vi "Add Item to Tree.vi"(6 "Display Text Override":string, 7 "Child only? (F)":bool, 8 "error in (no error)":errorcluster, 9 "Parent Tag":string, 10 "Data Item":refnum<class "Data Item.lvclass">, 11 "Tree Manager in":refnum<class "Tree Manager.lvclass">) -> (0 "error out":errorcluster, 2 "New Tag":string, 3 "Tree Manager out":refnum<class "Tree Manager.lvclass">)   [LabVIEW 2023, in "VILab.lvlib" / "Tree Manager.lvclass"]
uses:
  Tree Manager.lvclass
  Data Item.lvclass
  Tree Manager.lvclass/Tree Manager.ctl
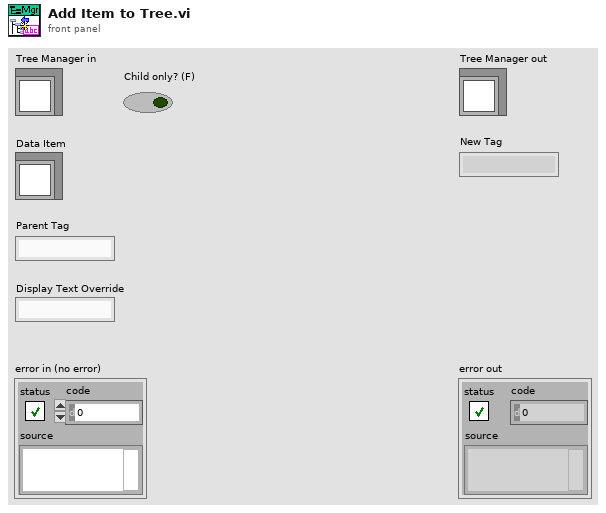
[diagram p1: front panel]
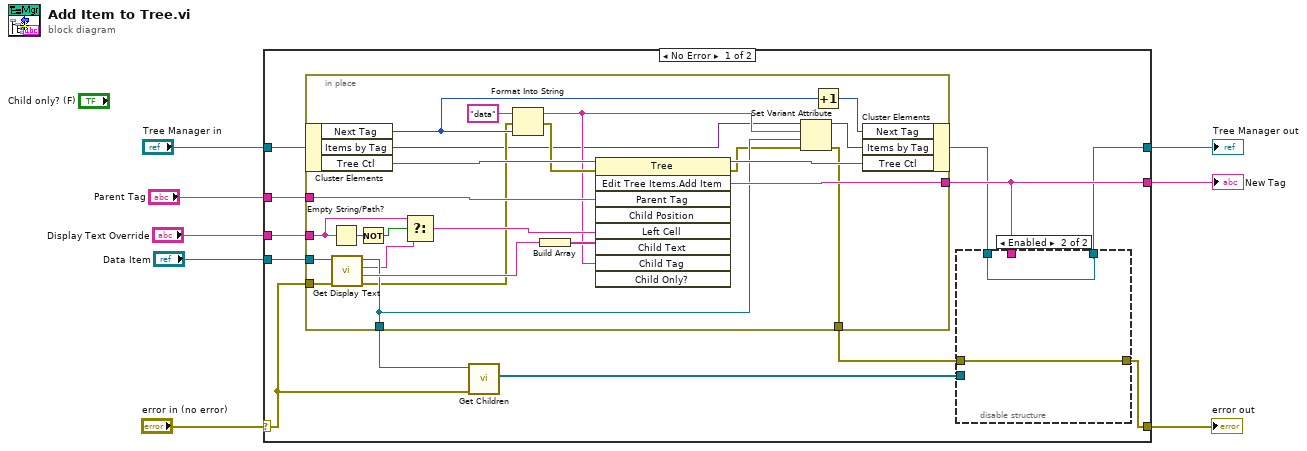
[diagram p0: block diagram]
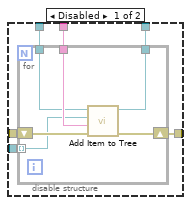
[diagram p2: hidden frame]
diagram:
  n1 = case shown="No Error" "error in (no error)" {
    selector: "error in (no error)" -> [w16 w60]
    tunnel: [w10 w60] -> w7
    tunnel: [w12 w59] -> w5
    tunnel: "Tree Manager in" -> [w19 w59]
    tunnel: "Data Item" -> [w20 _]
    tunnel: "Parent Tag" -> [w18 _]
    tunnel: [w15 _] -> w2
    tunnel: "Display Text Override" -> [w9 _]
    frame No Error {
      n2 = in-place {
        in-place-border: w20 -> [w58]
        in-place-border: w16 -> [w57]
        in-place-border: w18 -> [w55]
        in-place-border: [w47] -> w15
        in-place-border: [w46] -> w14
        in-place-border: [w45] -> w17
        in-place-border: w9 -> [w42]
        n3 = in-place-cluster #1(w19) -> ("Next Tag"=w49:u64, "Items by Tag"=w35:variant, "Tree Ctl"=w56:refnum<vi>)
        n4 = Empty String/Path?(string/path=w42) -> (empty?=w44:bool)
        n5 = call-dynamic "Get Display Text.vi"("error in (no error)"=w57, "Data Item in"=w58) -> ("error out"=w39:errorcluster, "Detail Text"=w54:string, "Display Name"=w41:string, "Data Item out"=w45:refnum<class "Data Item.lvclass">)  [unwired: 6 in]
        n6 = Not(x=w44) -> (.not. x?=w43:bool)
        n7 = Select(t=w42, s=w43, f=w41) -> (s? t:f=w40:string)
        n8 = Format Into String(initial string="data", error in=w39, w49) -> (resulting string=w36:string, error out=w38:errorcluster)  [unwired: 1 in]
        n9 = Build Array(w54) -> (w53:string[])
        n10 = invoke class="Tree" method="Edit Tree Items.Add Item"(reference=w56, error in=w38, "Parent Tag"=w55, "Left Cell"=w40, "Child Text"=w53, "Child Tag"=w36) -> (reference out=w52:refnum<vi>, error out=w37:errorcluster, "Edit Tree Items:Add Item"=w47:string)  [unwired: 3 in, 6 out]
        n11 = Set Variant Attribute(Variant=w35, name=w36, value=w45, error in=w37) -> (Variant out=w51:variant, error out=w46:errorcluster)  [unwired: 1 out]
        n12 = Increment(x=w49) -> (x+1=w50:u64)
        n13 = in-place-cluster #1("Next Tag"=w50, "Items by Tag"=w51, "Tree Ctl"=w52) -> (w13:refnum<class "Tree Manager.lvclass">)
      }
      n14 = call-dynamic "Get Children.vi"("error in (no error)"=w16, "Data Item in"=w17) -> ("Children"=w11:refnum<class "Data Item.lvclass">[])  [unwired: 7 in, 2 out]
      n15 = disable-structure shown="Enabled" {
        disable-tunnel: w15 -> [w26 _]
        disable-tunnel: w14 -> [w25 w34]
        disable-tunnel: w13 -> [w24 w33]
        disable-tunnel: [w23 w33] -> w12
        disable-tunnel: w11 -> [w22 _]
        disable-tunnel: [w21 w34] -> w10
        frame Disabled {
          n16 = for {
            tunnel: w26 -> [w32]
            shift-right: [w30] -> w21
            shift-left: w25 -> [w31]
            tunnel: w24 -> [w29]
            tunnel: [w28] -> w23
            tunnel: w22 -> [w27] mode=indexing
            n17 = call "Add Item to Tree.vi"("error in (no error)"=w31, "Parent Tag"=w32, "Data Item"=w27, "Tree Manager in"=w29) -> ("error out"=w30:errorcluster, "Tree Manager out"=w28:refnum<class "Tree Manager.lvclass">)  [unwired: 5 in, 1 out]
          }
        }
        frame Enabled {
        }
      }
    }
    frame Error {
    }
  }
  "error out" <- w7
  "Tree Manager out" <- w5
  "New Tag" <- w2
